vi "SetServiceClusterInputs.vi"(8 "error in":errorcluster, 10 "Properties":cluster{"Property":string, "Value":string}[](array[cluster]), 11 "Thing Info In":T2) -> (0 "error out":errorcluster, 3 "Thing Info Out":T2)   [LabVIEW 2015]
uses:
  <vilib>/httpClient/ClientHandle.ctl
  <vilib>/httpClient/POSTBuffer.vi
  <vilib>/httpClient/LabVIEWHTTPClient.lvlib
panel:
  out "Properties Array":cluster{"Property":string, "Value":string}[](array[cluster])
  in  "Value":string
  in  "Property":string
  out "final url":string
  out "reply body":string
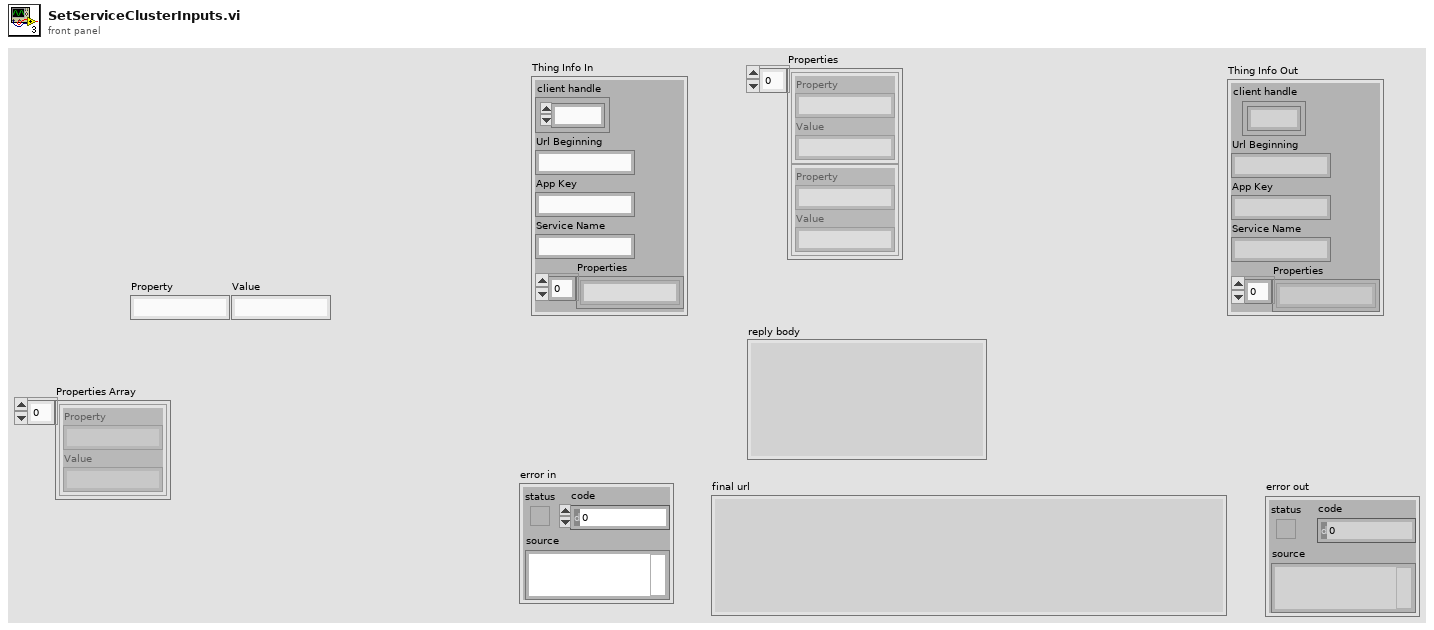
[diagram p1: front panel]
types:
  T1 = typedef "LabVIEWHTTPClient.lvlib/ClientHandle.ctl" = refnum<k1>
  T2 = cluster{"client handle":T1, "Url Beginning":string, "App Key":string, "Service Name":string, "Properties":string[]}
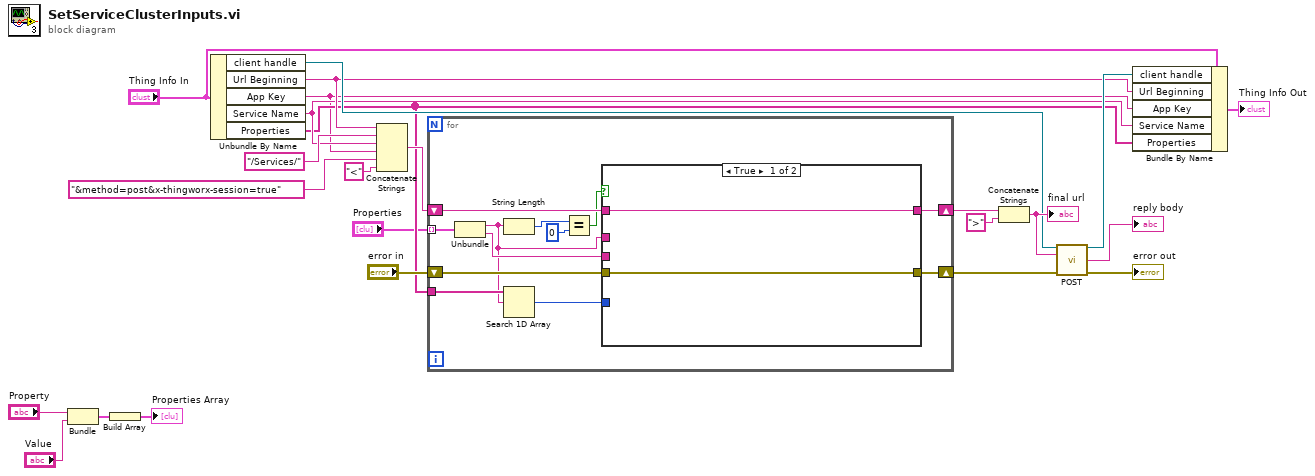
[diagram p0: block diagram]
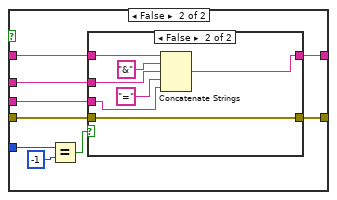
[diagram p2: hidden frame]
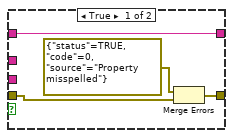
[diagram p3: hidden frame]
diagram:
  n1 = Bundle("Property"="Property", "Value"="Value") -> (w3:cluster{"Property":string, "Value":string})  [unwired: 1 in]
  n2 = Build Array(w3) -> (→"Properties Array":cluster{"Property":string, "Value":string}[])
  n3 = Unbundle By Name("Thing Info In") -> ("client handle"=w13:T1, "Url Beginning"=w11:string, "App Key"=w6:string, "Service Name"=w8:string, "Properties"=w7:string[])
  n4 = Concatenate Strings(w11, "/Services/" ("string"), w8, w6, "&method=post&x-thingworx-session=true" ("string"), "<" ("string")) -> (w20:string)
  n5 = for {
    shift-right: [w35] -> w19
    shift-left: w20 -> [w36]
    tunnel: w7 -> [w27]
    shift-right: [w30] -> w14
    shift-left: "error in" -> [w31]
    tunnel: "Properties" -> [w29] mode=indexing
    n6 = Unbundle(w29) -> ("Property"=w25:string, "Value"=w26:string)
    n7 = String Length(string=w25) -> (length=w28:i32)
    n8 = Search 1D Array(1D array=w27, element=w25) -> (index of element=w34:i32)  [unwired: 1 in]
    n9 = Equal?(x=w28, y=0) -> (x = y?=w32:bool)
    n10 = case shown="True" w32 {
      tunnel: w36 -> [w38 w47]
      tunnel: [w38 w46] -> w35
      tunnel: w34 -> [_ w44]
      tunnel: w31 -> [w37 w42]
      tunnel: [w37 w41] -> w30
      tunnel: w26 -> [_ w40]
      tunnel: w25 -> [_ w39]
      frame True {
      }
      frame False {
        n11 = Equal?(x=w44, y=-1) -> (x = y?=w43:bool)
        n12 = case shown="False" w43 {
          tunnel: w47 -> [w48 w58]
          tunnel: [w48 w57] -> w46
          tunnel: w42 -> [w51 w54]
          tunnel: [w49 w54] -> w41
          tunnel: w40 -> [_ w53]
          tunnel: w39 -> [_ w52]
          frame True {
            n13 = Merge Errors(errorcluster {"status"=TRUE, "code"=0, "source"="Property misspelled"} ("error in"), w51) -> (w49:errorcluster)
          }
          frame False {
            n14 = Concatenate Strings(w58, "&" ("string"), w52, "=" ("string"), w53) -> (w57:string)
          }
        }
      }
    }
  }
  n15 = Concatenate Strings(w19, ">" ("string")) -> (w18:string)
  "final url" <- w18
  n16 = call-poly <vilib>:"POST.vi"("client handle"=w13, "url"=w18, "error in (no error)"=w14) -> ("client handle out"=w12:T1, "body"=→"reply body":string, "error out"=→"error out":errorcluster)  [unwired: 9 in, 1 out]
  n17 = Bundle By Name(cluster="Thing Info In", "client handle"=w12, "Url Beginning"=w11, "App Key"=w6, "Service Name"=w8, "Properties"=w7) -> (→"Thing Info Out":T2)
